vi "Init.vi"(8 "error in (no error)":errorcluster, 10 "IConfigure":refnum<class "IConfigure.lvclass">, 11 "Fgen Base in":refnum<class "Fgen Base.lvclass">) -> (0 "error out":errorcluster, 3 "Fgen Base out":refnum<class "Fgen Base.lvclass">)   [LabVIEW 2023, in "Fgen Base.lvclass"]
uses:
  Fgen Base.lvclass
  Fgen Base.lvclass/Fgen Base.ctl
  Interfaces/IConfigure/IConfigure.lvclass
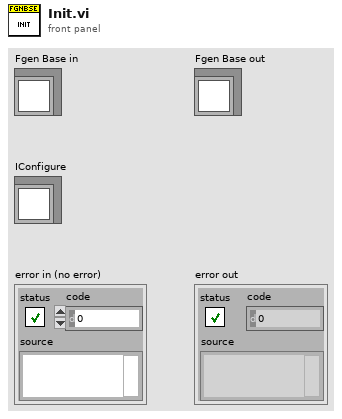
[diagram p1: front panel]
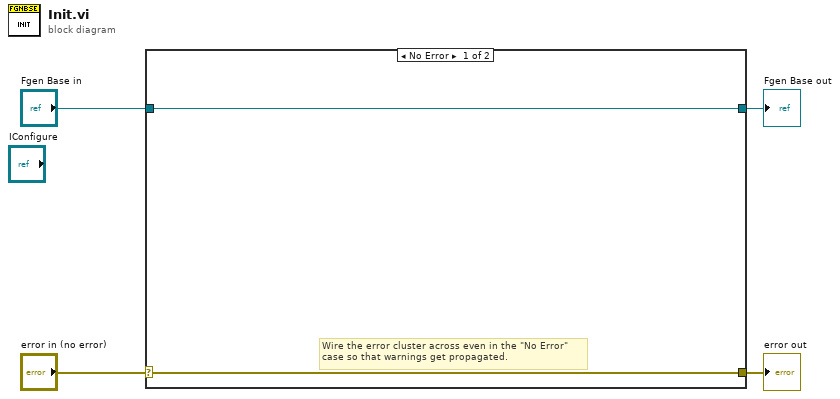
[diagram p0: block diagram]
diagram:
  n1 = case shown="No Error" "error in (no error)" {
    selector: "error in (no error)" -> [w5 w8]
    tunnel: [w5 w8] -> w3
    tunnel: [w6 w7] -> w1
    tunnel: "Fgen Base in" -> [w6 w7]
    frame No Error {
      # "Wire the error cluster across even in the \"No Error\"\ncase so that warnings get propagated."
    }
    frame Error {
    }
  }
  "error out" <- w3
  "Fgen Base out" <- w1
